vi "Example Convex Hul.vi"() -> ()   [LabVIEW 2015]
uses:
  <vilib>/numeric/Random Number (Range) DBL.vi
  LV QHull/QHull.lvlib
  <vilib>/Math Plots/3D Math Plots/3D Scatter/3D Scatter Datatype/3D Scatter Datatype.lvclass
  <vilib>/Math Plots/3D Math Plots/3D Scatter/3D Scatter Datatype/Public/Plot Helper (Vector).vi
  <vilib>/Math Plots/3D Math Plots/3D Scatter/3D Scatter XCtrl/3D Scatter.xctl
panel:
  out "3D Scatter":refnum<class "3D Plot Datatype.lvclass">[](xcontrol)
  out "XY Graph":cluster{cluster{"number":dbl, "number":dbl}[]}[](graph)
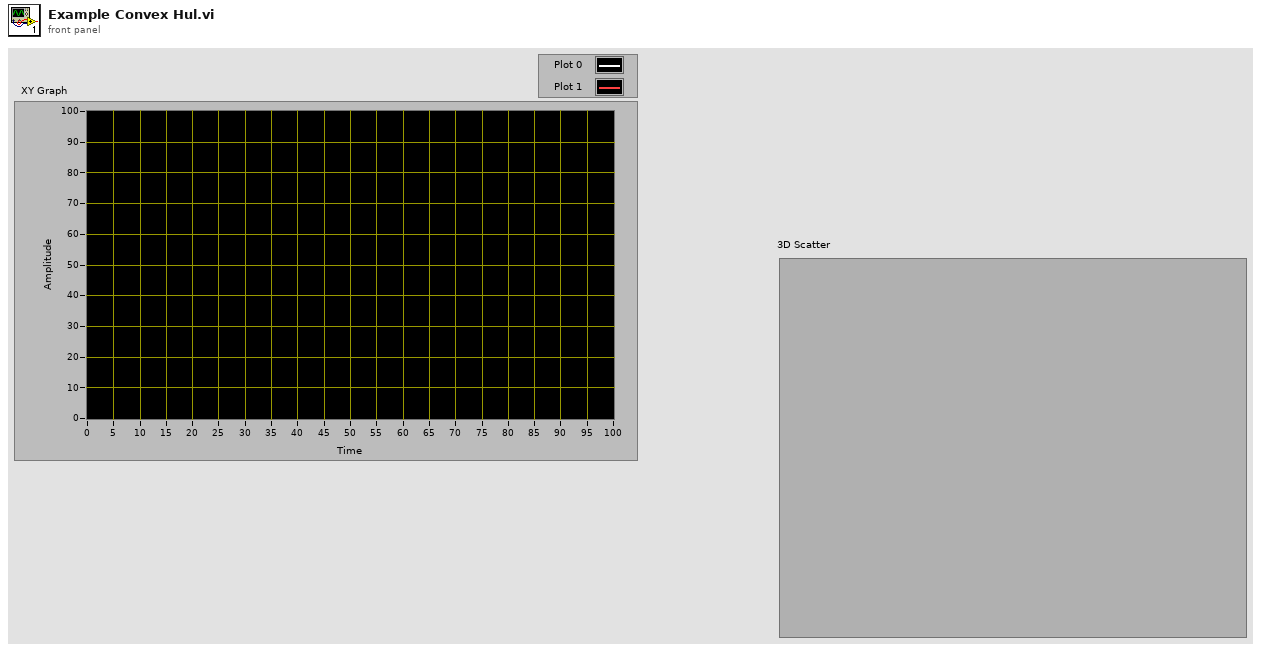
[diagram p1: front panel]
types:
  T1 = cluster{"number":dbl, "number":dbl, "number":dbl}
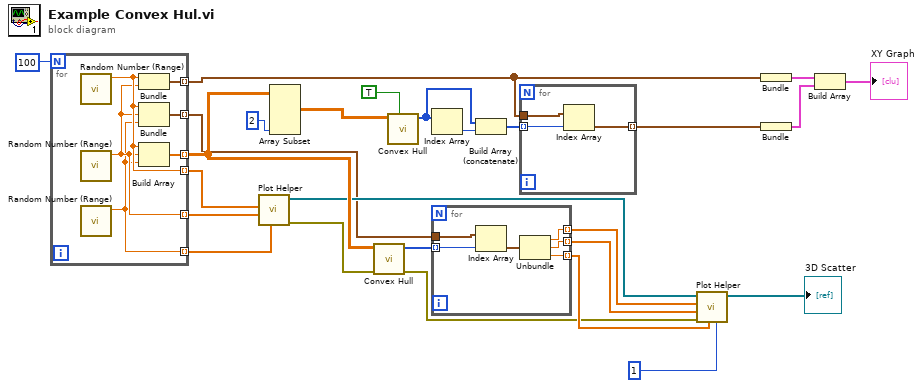
[diagram p0: block diagram]
diagram:
  n1 = for {
    N: 100 -> [_]
    tunnel: [w32] -> w14 mode=indexing
    tunnel: [w31] -> w21 mode=indexing
    tunnel: [w30] -> w7 mode=indexing
    tunnel: [w29] -> w12 mode=indexing
    tunnel: [w28] -> w11 mode=indexing
    tunnel: [w27] -> w10 mode=indexing
    n2 = call-poly <vilib>:"Random Number (Range).vi"() -> ("number"=w29:dbl)  [unwired: 11 in]
    n3 = call-poly <vilib>:"Random Number (Range).vi"() -> ("number"=w28:dbl)  [unwired: 11 in]
    n4 = call-poly <vilib>:"Random Number (Range).vi"() -> ("number"=w27:dbl)  [unwired: 11 in]
    n5 = Bundle("number"=w29, "number"=w28) -> (w31:cluster{"number":dbl, "number":dbl})  [unwired: 1 in]
    n6 = Bundle("number"=w29, "number"=w28, "number"=w27) -> (w30:T1)  [unwired: 1 in]
    n7 = Build Array(w29, w28, w27) -> (w32:dbl[])
  }
  n8 = call-poly <vilib>:"Plot Helper.vi"("z vector"=w10, "y vector"=w11, "x vector"=w12) -> ("error out"=w2:errorcluster, "3D Plot lvclass Array out"=w9:refnum<class "3D Plot Datatype.lvclass">[])  [unwired: 3 in, 4 out]
  n9 = Array Subset(array=w14, length (col)=2 ("length")) -> (w16:dbl[][])  [unwired: 3 in]
  n10 = call "Convex Hull.vi"("error in (no error)"=w2, "points"=w14) -> ("error out"=w1:errorcluster, "Simplex Indices"=w13:i32[])  [unwired: 6 in, 2 out]
  n11 = call "Convex Hull.vi"("Sort CW in 2D"=TRUE, "points"=w16) -> ("Simplex Indices"=w18:i32[])  [unwired: 6 in, 3 out]
  n12 = Index Array(array=w18) -> (element=w17:i32)  [unwired: 1 in]
  n13 = for {
    tunnel: w13 -> [w37] mode=indexing
    tunnel: w7 -> [w38]
    tunnel: [w35] -> w6 mode=indexing
    tunnel: [w34] -> w5 mode=indexing
    tunnel: [w33] -> w4 mode=indexing
    n14 = Index Array(array=w38, index=w37) -> (element=w36:T1)
    n15 = Unbundle(w36) -> ("number"=w35:dbl, "number"=w34:dbl, "number"=w33:dbl)
  }
  n16 = Build Array (concatenate)(w18, w17) -> (w19:i32[])
  n17 = for {
    tunnel: [w40] -> w22 mode=indexing
    tunnel: w21 -> [w41]
    tunnel: w19 -> [w39] mode=indexing
    n18 = Index Array(array=w41, index=w39) -> (element=w40:cluster{"number":dbl, "number":dbl})
  }
  n19 = call-poly <vilib>:"Plot Helper.vi"("Plot ID"=1, "z vector"=w4, "error in (no error)"=w1, "y vector"=w5, "x vector"=w6, "3D Plot lvclass Array in"=w9) -> ("3D Plot lvclass Array out"=→"3D Scatter":refnum<class "3D Plot Datatype.lvclass">[])  [unwired: 5 out]
  n20 = Bundle(w21) -> (w25:cluster{cluster{"number":dbl, "number":dbl}[]})  [unwired: 1 in]
  n21 = Bundle(w22) -> (w23:cluster{cluster{"number":dbl, "number":dbl}[]})  [unwired: 1 in]
  n22 = Build Array(w25, w23) -> (→"XY Graph":cluster{cluster{"number":dbl, "number":dbl}[]}[])
